vi "mxwScript_Cmnd2Str_setConnectorPane.vi"(8 "error in (no error)":errorcluster, 11 "data":variant) -> (0 "error out":errorcluster, 3 "outputString":string)   [LabVIEW 2020]
uses:
  codeGenAPISupport.llb/cgAPI_mxwScript_ConnectorPane.ctl
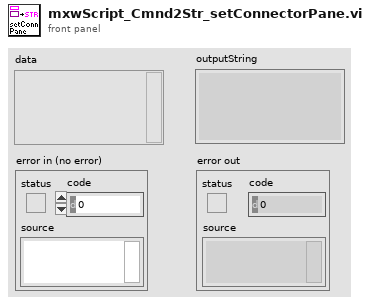
[diagram p1: front panel]
types:
  T1 = typedef "cgAPI_mxwScript_ConnectorPane.ctl" = cluster{"pane":u32, "rotation":string}
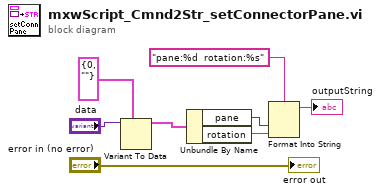
[diagram p0: block diagram]
diagram:
  n1 = Variant To Data(type=T1 {"pane"=0, "rotation"=""} ("connectorPane"), Variant="data") -> (data=w6:T1)  [unwired: 1 in, 1 out]
  n2 = Unbundle By Name(w6) -> ("pane"=w3:u32, "rotation"=w4:string)
  n3 = Format Into String(format string="pane:%d  rotation:%s", w3, w4) -> (resulting string=→"outputString":string)  [unwired: 2 in, 1 out]
  "error out" <- "error in (no error)"
